vi "로또번호 생성기.vi"() -> ()   [LabVIEW 2018]
panel:
  out "배열":dbl[](array[numeric])
  out "행운 번호":dbl
  in  "번호생성":bool
  in  "정지 버튼":bool
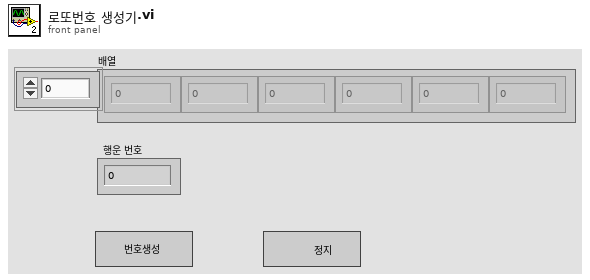
[diagram p1: front panel]
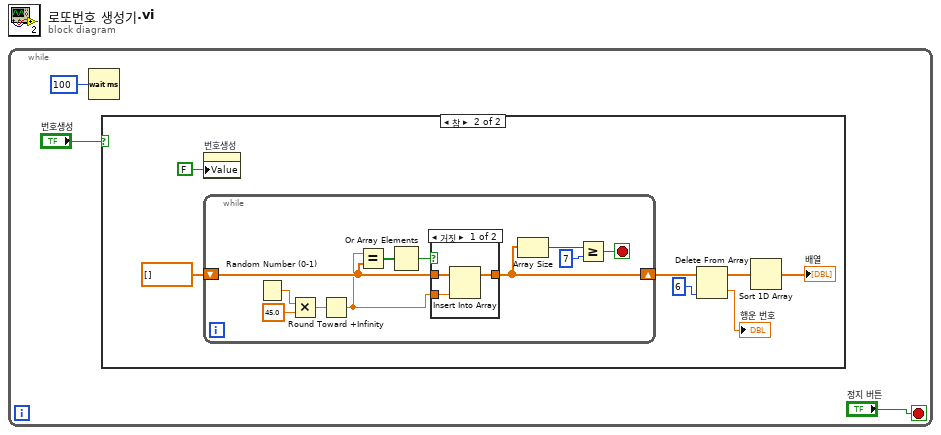
[diagram p0: block diagram]
diagram:
  n1 = while {
    stop <- "정지 버튼" stop-if-true
    n2 = Wait (ms)(milliseconds to wait=u32 100 ("대기 시간 (ms)")) -> ()  [unwired: 1 out]
    n3 = case shown="참" "번호생성" {
      frame False {
      }
      frame True {
        n4 = property on="번호생성" class="Bool (엄격한)"("Value"=FALSE ("번호생성")) -> ()  [unwired: 2 in, 2 out]
        n5 = while {
          shift-right: [w14] -> w9
          shift-left: dbl[] [] -> [w16]
          stop <- w12 stop-if-true
          n6 = Random Number (0-1)() -> (number: 0 to 1=w21:dbl)
          n7 = Multiply(x=w21, y=45.0) -> (x*y=w19:dbl)
          n8 = Round Toward +Infinity(x=w19) -> (ceil(x): smallest int >= x=w15:dbl)
          n9 = Equal?(x=w15, y=w16) -> (x = y?=w18:bool[])
          n10 = Or Array Elements(Boolean array=w18) -> (logical OR=w17:bool)
          n11 = case shown="거짓" w17 {
            tunnel: w16 -> [w24 w25]
            tunnel: w15 -> [w23 _]
            tunnel: [w22 w25] -> w14
            frame False {
              n12 = Insert Into Array(array=w24, new element=w23) -> (w22:dbl[])  [unwired: 1 in]
            }
            frame True {
            }
          }
          n13 = Array Size(array=w14) -> (size(s)=w13:i32)
          n14 = Greater Or Equal?(x=w13, y=7) -> (x >= y?=w12:bool)
        }
        n15 = Delete From Array(array=w9, index=6 ("인덱스")) -> (deleted portion=→"행운 번호":dbl, array with subset deleted=w6:dbl[])  [unwired: 1 in]
        n16 = Sort 1D Array(array=w6) -> (sorted array=→"배열":dbl[])
      }
    }
  }
